vi "U6 eDAC Example.vi"() -> (0 "error out":errorcluster)   [LabVIEW 2021]
panel:
  in  "Address":string="1"
  in  "FirstFound":bool=TRUE
  in  "Channel":i32
  out "Error Message":string
  in  "Voltage":dbl format="%.3f"
  # "Sets 1 analog output using the UD easy function eDAC."
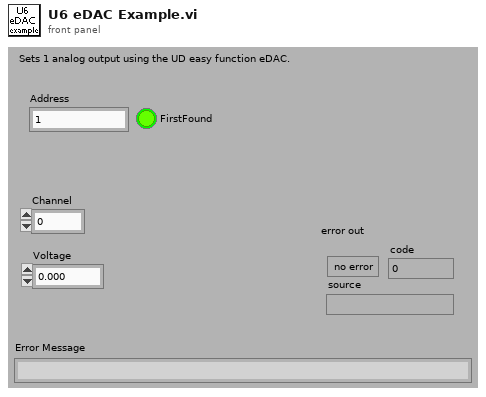
[diagram p1: front panel]
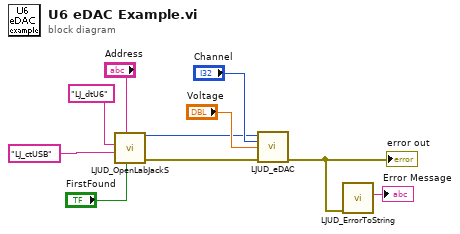
[diagram p0: block diagram]
diagram:
  n1 = call "LJUD_OpenLabJackS.vi"("FirstFound"="FirstFound", "Address"="Address", "ConnectionType"="LJ_ctUSB", "DeviceType"="LJ_dtU6") -> ("error out"=w2:errorcluster, "Handle"=w3:i32)  [unwired: 5 in, 1 out]
  n2 = call "LJUD_eDAC.vi"("Handle In"=w3, "Channel"="Channel", "Voltage"="Voltage", "error in"=w2) -> ("error out"=w9:errorcluster)  [unwired: 10 in, 1 out]
  "error out" <- w9
  n3 = call "LJUD_ErrorToString.vi"("error in"=w9) -> ("String"=→"Error Message":string)  [unwired: 10 in]
